vi "End Section.vi"(8 "error in (no error)":errorcluster {"code" format="Error %.0f"}, 10 "Section":string, 11 "VIDoc Parser In":refnum<class "VIDoc Parser.lvclass">) -> (0 "error out":errorcluster {"code" format="Error %.0f"}, 3 "VIDoc Parser Out":refnum<class "VIDoc Parser.lvclass">)   [LabVIEW 2023, in "VIDoc Parsing.lvlib" / "VIDoc Parser.lvclass"]
uses:
  VIDoc Parser.lvclass
  VIDoc Parser.lvclass/VIDoc Parser.ctl
  UI Interaction/UI Interaction.lvclass
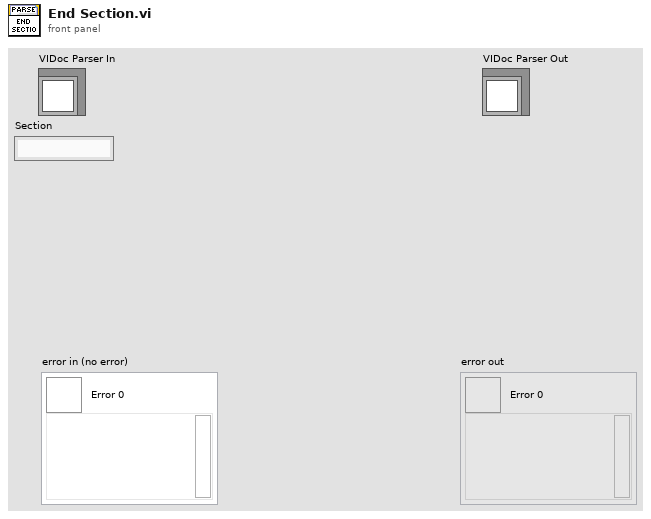
[diagram p1: front panel]
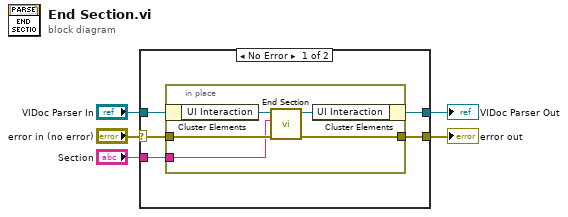
[diagram p0: block diagram]
diagram:
  n1 = case shown="No Error" "error in (no error)" {
    selector: "error in (no error)" -> [w8 w17]
    tunnel: [w7 w17] -> w4
    tunnel: [w10 w16] -> w2
    tunnel: "VIDoc Parser In" -> [w9 w16]
    tunnel: "Section" -> [w6 _]
    frame No Error {
      n2 = in-place {
        in-place-border: w8 -> [w13]
        in-place-border: [w12] -> w7
        in-place-border: w6 -> [w11]
        n3 = in-place-cluster #1(w9) -> ("UI Interaction"=w15:refnum<class "UI Interaction.lvclass">)
        n4 = call-dynamic "End Section.vi"("error in (no error)"=w13, "Section"=w11, "UI Interaction in"=w15) -> ("error out"=w12:errorcluster, "UI Interaction out"=w14:refnum<class "UI Interaction.lvclass">)  [unwired: 7 in]
        n5 = in-place-cluster #1("UI Interaction"=w14) -> (w10:refnum<class "VIDoc Parser.lvclass">)
      }
    }
    frame Error {
    }
  }
  "error out" <- w4
  "VIDoc Parser Out" <- w2
